vi "traitement cam 33.vi"() -> (11 "Couleur carré 11 (1,9)":string[](array[string]), 13 "Couleur carré 10  (1,8)":string[](array[string]), 14 "Couleur carré 4 (2,1)":string[](array[string]), 15 "Couleur carré 9 (1,7)":string[](array[string]), 16 "Couleur carré 3 (2,4)":string[](array[string]), 17 "Couleur carré 12 (1,4)":string[](array[string]), 18 "Couleur carré 2 (2,7)":string[](array[string]), 19 "Image Out":T2(plugin-control), 20 "Couleur carré 1 (2,8)":string[](array[string]), 22 "Couleur carré 5 (6,4)":string[](array[string]), 23 "Couleur carré 6 (6,1)":string[](array[string]), 24 "Couleur carré 7 (6,2)":string[](array[string]), 25 "Couleur carré 8 (6,3)":string[](array[string]), 27 "error out":errorcluster)   [LabVIEW 2019]
uses:
  <vilib>/vision/Classification.llb/IMAQ Classifier Read Options.ctl
  <vilib>/vision/NI_Vision_Development_Module.lvlib
panel:
  in  "ROI Carré 1":T1={"Global Rectangle"=[636, 369, 672, 405], "Contours"=[{"ID"=enum."External", "Type"=3, "Coordinates"=[636, 369, 672, 405]}]} {"Contours"."Type" items=["No Selection", "Point", "Line", "Rectangle", "Oval", "Polygon", "Freehand Region", "Annulus", "Unused2", "Unused3", "Broken Line", "Freehand Line", "Rotated Rectangle"]}
  in  "error in":errorcluster
  in  "ROI Carré 12":T1={"Global Rectangle"=[636, 369, 672, 405], "Contours"=[{"ID"=enum."External", "Type"=3, "Coordinates"=[636, 369, 672, 405]}]} {"Contours"."Type" items=["No Selection", "Point", "Line", "Rectangle", "Oval", "Polygon", "Freehand Region", "Annulus", "Unused2", "Unused3", "Broken Line", "Freehand Line", "Rotated Rectangle"]}
  in  "ROI Carré 11":T1={"Global Rectangle"=[636, 369, 672, 405], "Contours"=[{"ID"=enum."External", "Type"=3, "Coordinates"=[636, 369, 672, 405]}]} {"Contours"."Type" items=["No Selection", "Point", "Line", "Rectangle", "Oval", "Polygon", "Freehand Region", "Annulus", "Unused2", "Unused3", "Broken Line", "Freehand Line", "Rotated Rectangle"]}
  in  "ROI Carré 10":T1={"Global Rectangle"=[636, 369, 672, 405], "Contours"=[{"ID"=enum."External", "Type"=3, "Coordinates"=[636, 369, 672, 405]}]} {"Contours"."Type" items=["No Selection", "Point", "Line", "Rectangle", "Oval", "Polygon", "Freehand Region", "Annulus", "Unused2", "Unused3", "Broken Line", "Freehand Line", "Rotated Rectangle"]}
  in  "ROI Carré 9":T1={"Global Rectangle"=[636, 369, 672, 405], "Contours"=[{"ID"=enum."External", "Type"=3, "Coordinates"=[636, 369, 672, 405]}]} {"Contours"."Type" items=["No Selection", "Point", "Line", "Rectangle", "Oval", "Polygon", "Freehand Region", "Annulus", "Unused2", "Unused3", "Broken Line", "Freehand Line", "Rotated Rectangle"]}
  in  "ROI Carré 8":T1={"Global Rectangle"=[636, 369, 672, 405], "Contours"=[{"ID"=enum."External", "Type"=3, "Coordinates"=[636, 369, 672, 405]}]} {"Contours"."Type" items=["No Selection", "Point", "Line", "Rectangle", "Oval", "Polygon", "Freehand Region", "Annulus", "Unused2", "Unused3", "Broken Line", "Freehand Line", "Rotated Rectangle"]}
  in  "ROI Carré 7":T1={"Global Rectangle"=[636, 369, 672, 405], "Contours"=[{"ID"=enum."External", "Type"=3, "Coordinates"=[636, 369, 672, 405]}]} {"Contours"."Type" items=["No Selection", "Point", "Line", "Rectangle", "Oval", "Polygon", "Freehand Region", "Annulus", "Unused2", "Unused3", "Broken Line", "Freehand Line", "Rotated Rectangle"]}
  in  "ROI Carré 6":T1={"Global Rectangle"=[636, 369, 672, 405], "Contours"=[{"ID"=enum."External", "Type"=3, "Coordinates"=[636, 369, 672, 405]}]} {"Contours"."Type" items=["No Selection", "Point", "Line", "Rectangle", "Oval", "Polygon", "Freehand Region", "Annulus", "Unused2", "Unused3", "Broken Line", "Freehand Line", "Rotated Rectangle"]}
  in  "ROI Carré 5":T1={"Global Rectangle"=[636, 369, 672, 405], "Contours"=[{"ID"=enum."External", "Type"=3, "Coordinates"=[636, 369, 672, 405]}]} {"Contours"."Type" items=["No Selection", "Point", "Line", "Rectangle", "Oval", "Polygon", "Freehand Region", "Annulus", "Unused2", "Unused3", "Broken Line", "Freehand Line", "Rotated Rectangle"]}
  in  "ROI Carré 4":T1={"Global Rectangle"=[636, 369, 672, 405], "Contours"=[{"ID"=enum."External", "Type"=3, "Coordinates"=[636, 369, 672, 405]}]} {"Contours"."Type" items=["No Selection", "Point", "Line", "Rectangle", "Oval", "Polygon", "Freehand Region", "Annulus", "Unused2", "Unused3", "Broken Line", "Freehand Line", "Rotated Rectangle"]}
  in  "ROI Carré 3":T1={"Global Rectangle"=[636, 369, 672, 405], "Contours"=[{"ID"=enum."External", "Type"=3, "Coordinates"=[636, 369, 672, 405]}]} {"Contours"."Type" items=["No Selection", "Point", "Line", "Rectangle", "Oval", "Polygon", "Freehand Region", "Annulus", "Unused2", "Unused3", "Broken Line", "Freehand Line", "Rotated Rectangle"]}
  in  "ROI Carré 2":T1={"Global Rectangle"=[636, 369, 672, 405], "Contours"=[{"ID"=enum."External", "Type"=3, "Coordinates"=[636, 369, 672, 405]}]} {"Contours"."Type" items=["No Selection", "Point", "Line", "Rectangle", "Oval", "Polygon", "Freehand Region", "Annulus", "Unused2", "Unused3", "Broken Line", "Freehand Line", "Rotated Rectangle"]}
  # "C\nE\nN\nT\nR\nE\n\nJ\nA\nU\nN\nE\n\nBAS"
  # "C\nE\nN\nT\nR\nE\n\nV\nE\nR\nT\n\nG"
  # "C\nE\nN\nT\nR\nE\n\nR\nO\nU\nG\nE\n\nD"
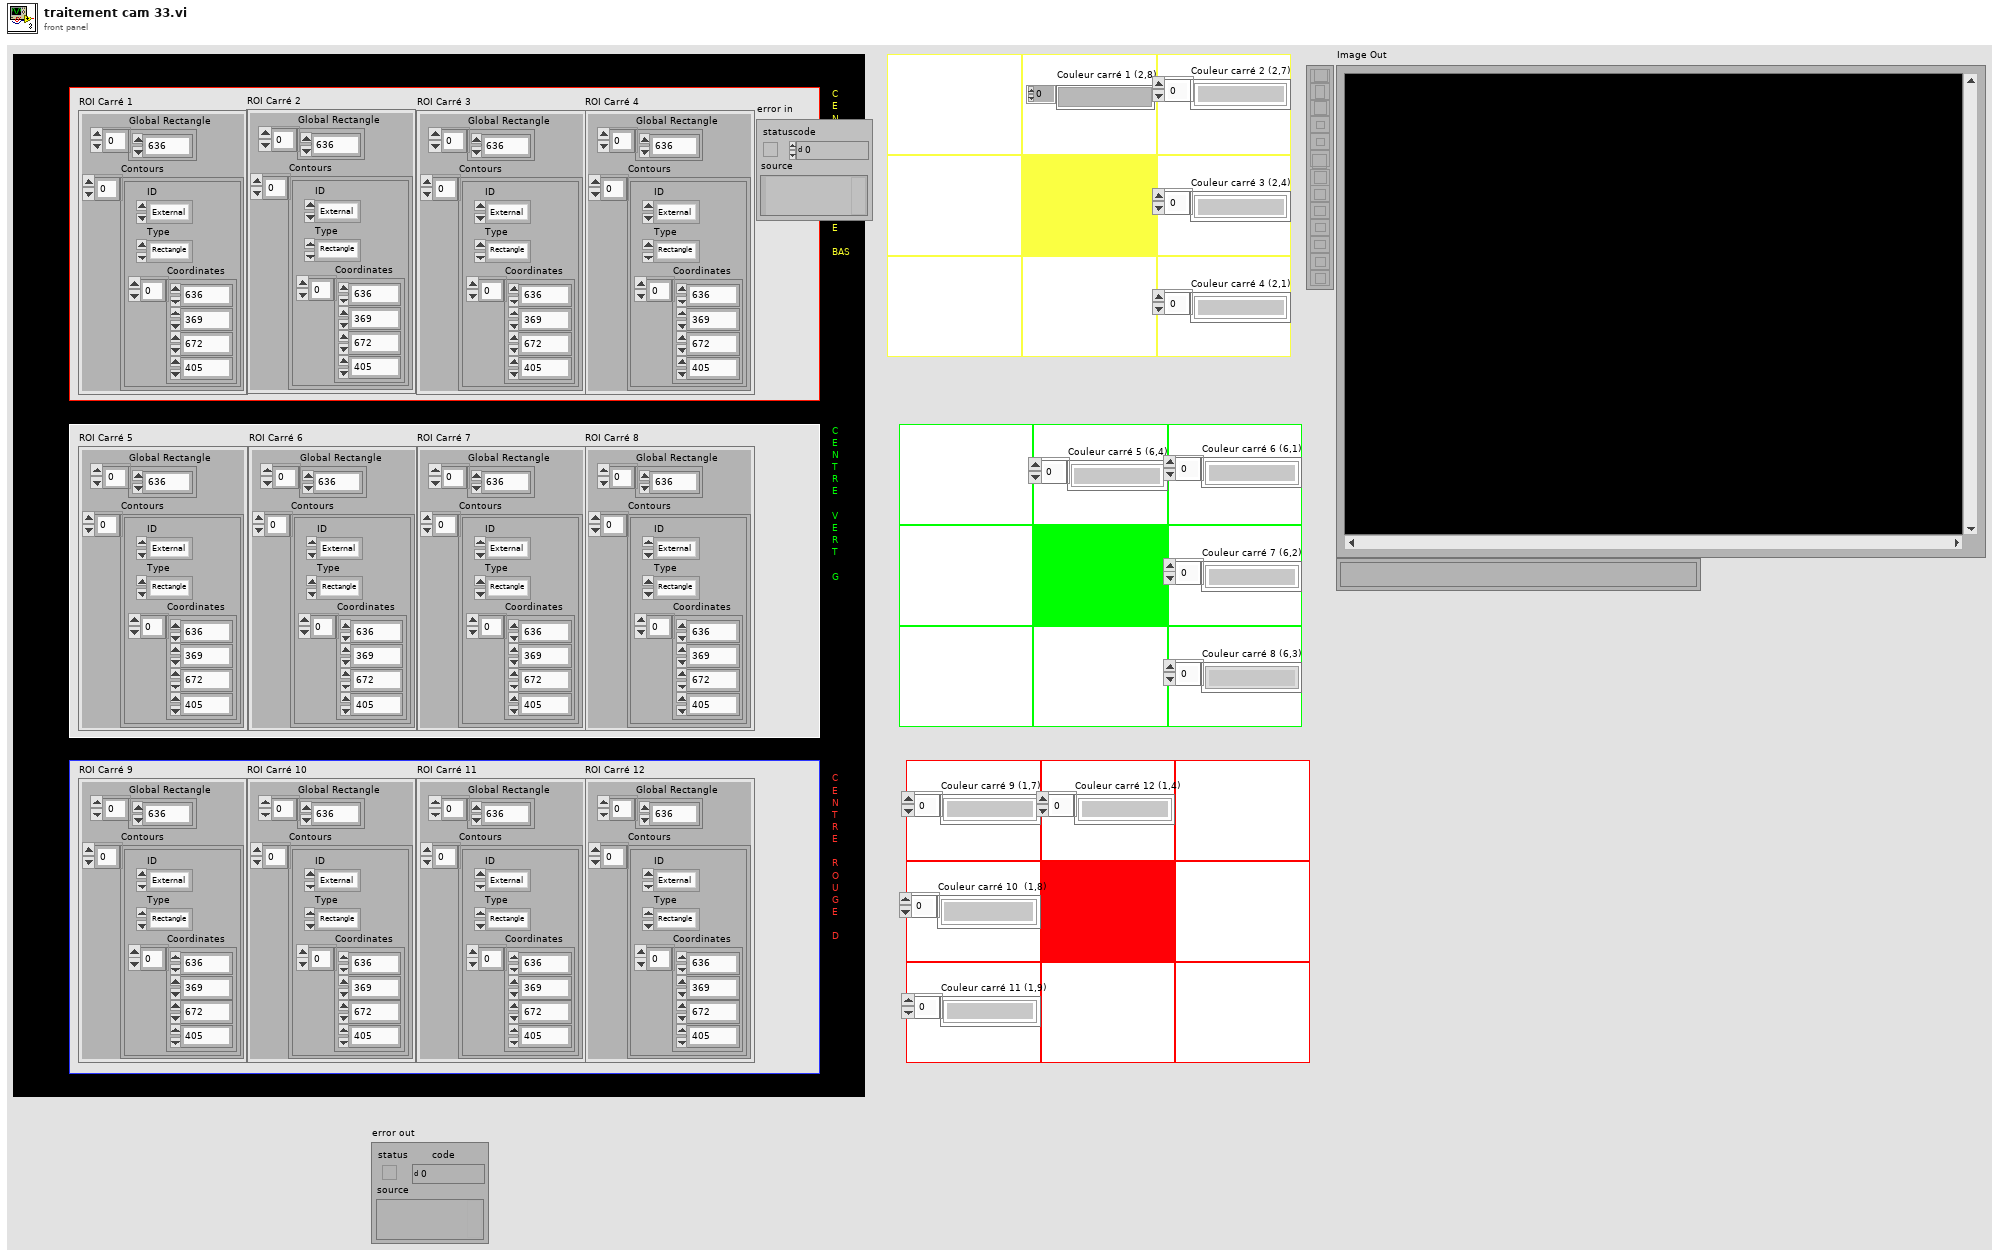
[diagram p1: front panel]
types:
  T1 = cluster{"Global Rectangle":i32[], "Contours":cluster{"ID":enum32{"External", "Internal"}, "Type":u32, "Coordinates":i32[]}[]}
  T2 = typedef "IMAQ Image.ctl" = refnum<image>
  T3 = typedef "IMAQ Classifier Read Options.ctl" = i32
  T4 = typedef "IMAQ Classifier Session.ctl" = refnum<k1>
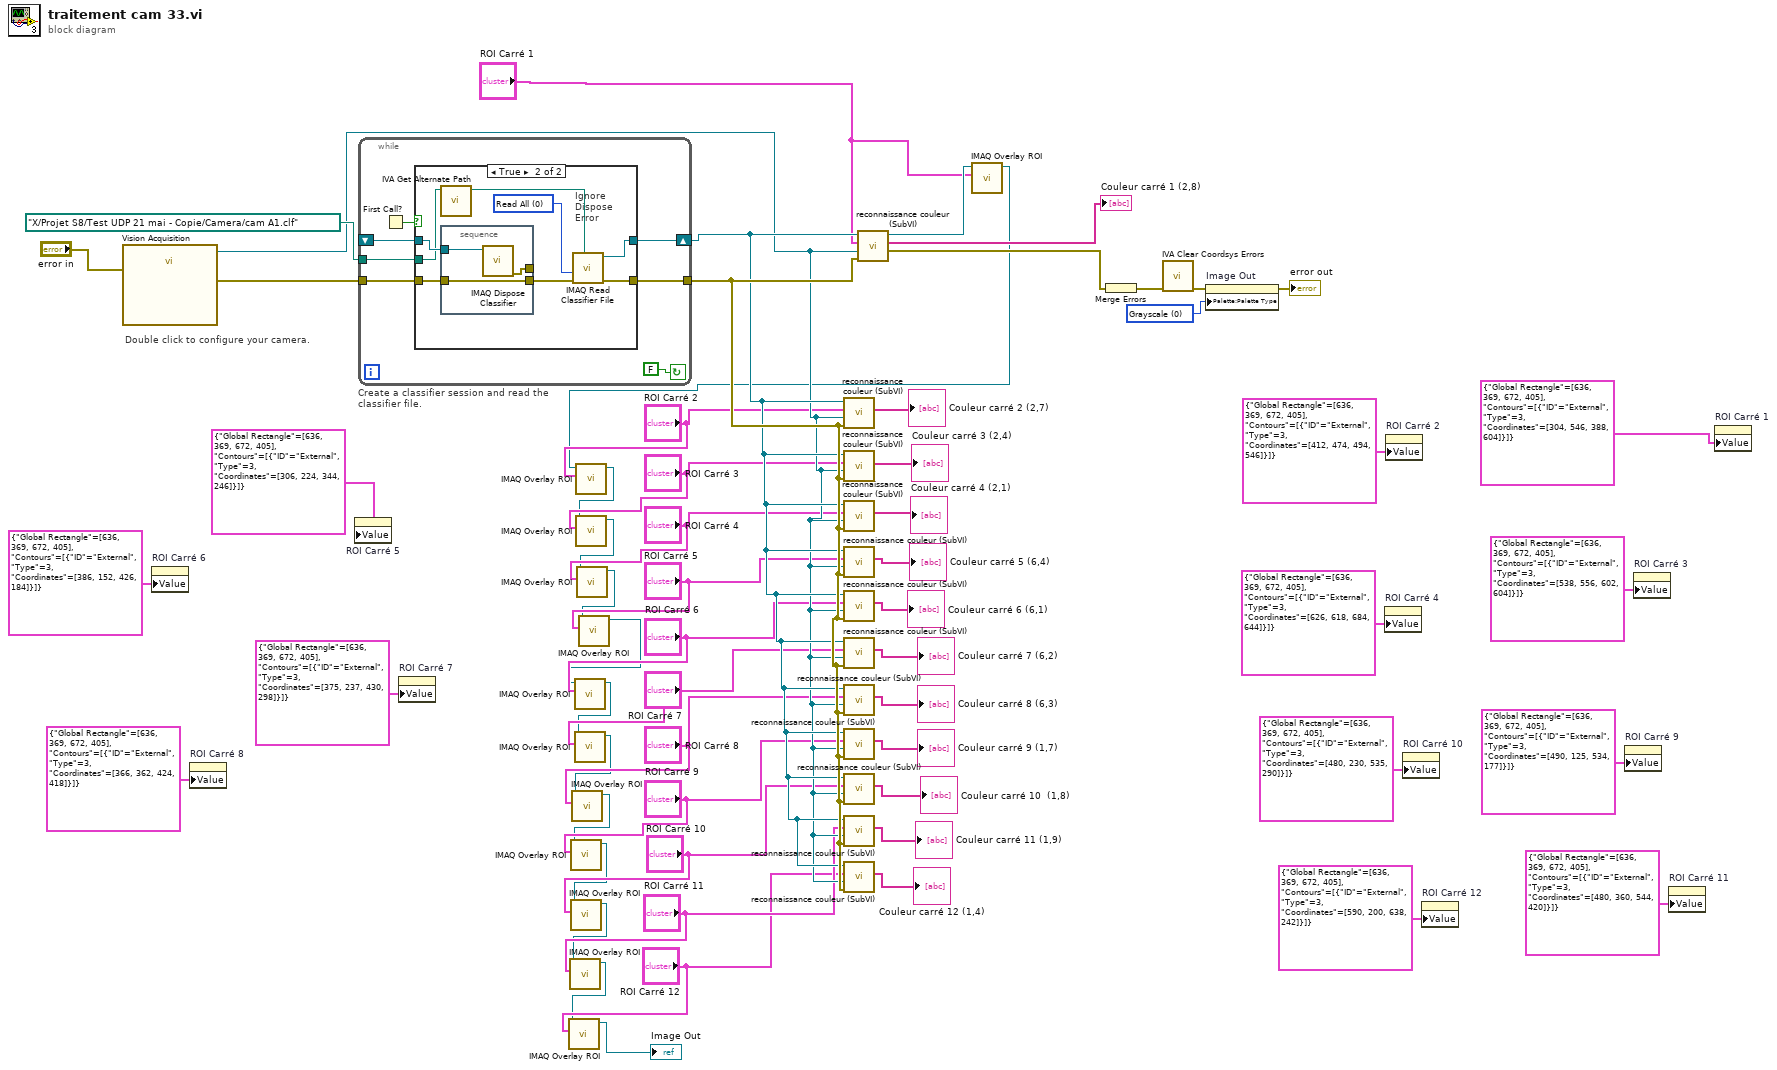
[diagram p0: block diagram]
diagram:
  w53 = u32 0 items=["Grayscale", "Binary", "Gradient", "Rainbow", "Temperature", "User Defined", "Binary 16 Bit", "Gradient 16 Bit", "Rainbow 16 Bit", "Temperature 16 Bit", "User Defined 16 Bit"] ("Palette Type")
  # "Double click to configure your camera."
  n1 = call "Vision Acquisition"("error in"="error in") -> ("Image Out"=w39:T2, "error out"=w58:errorcluster)  [unwired: 25 in]
  n2 = property on="ROI Carré 6" class="Clust (strict)"("Value"=T1 {"Global Rectangle"=[636, 369, 672, 405], "Contours"=[{"ID"=enum."External", "Type"=3, "Coordinates"=[386, 152, 426, 184]}]} ("ROI Carré 6")) -> ()  [unwired: 2 in, 2 out]
  n3 = property on="ROI Carré 8" class="Clust (strict)"("Value"=T1 {"Global Rectangle"=[636, 369, 672, 405], "Contours"=[{"ID"=enum."External", "Type"=3, "Coordinates"=[366, 362, 424, 418]}]} ("ROI Carré 8")) -> ()  [unwired: 2 in, 2 out]
  n4 = property on="ROI Carré 5" class="Clust (strict)"("Value"=T1 {"Global Rectangle"=[636, 369, 672, 405], "Contours"=[{"ID"=enum."External", "Type"=3, "Coordinates"=[306, 224, 344, 246]}]} ("ROI Carré 5")) -> ()  [unwired: 2 in, 2 out]
  n5 = while "Create a classifier session and read the classifier file." {
    shift-right: [w67] -> w50
    shift-left: _ -> [w66]
    tunnel: w58 -> [w64]
    tunnel: [w63] -> w51
    tunnel: path "X:/Projet S8/Test UDP 21 mai - Copie/Camera/cam A1.clf" ("File Path") -> [w62]
    stop <- FALSE continue-if-true
    n6 = First Call?() -> (First Call?: T/F=w61:bool)
    n7 = case shown="True" w61 {
      tunnel: [w69 w76] -> w67
      tunnel: w66 -> [w69 w74]
      tunnel: w64 -> [w68 w73]
      tunnel: [w68 w75] -> w63
      tunnel: w62 -> [_ w71]
      frame False {
      }
      frame True {
        w77 = T3 0 items=["Read All", "Add Samples, Do Not Change Options", "Read Options, Do Not Add Samples"] ("Read Options")
        # "Ignore Dispose Error"
        n8 = call <vilib>:"IVA Get Alternate Path.vi"("Path In"=w71) -> ("Path Out"=w70:path)  [unwired: 10 out]
        n9 = stacked-sequence {
          tunnel: w74 -> [w80]
          tunnel: w73 -> [w79]
          tunnel: [w79] -> w72
          tunnel: [w78] -> _
          frame #0 {
            n10 = call "IMAQ Dispose Classifier"("Classifier Session"=w80) -> ("error out"=w78:errorcluster)  [unwired: 1 in, 9 out]
          }
        }
        n11 = call "IMAQ Read Classifier File"("File Path"=w70, "error in (no error)"=w72, "Read Options"=w77) -> ("error out"=w75:errorcluster, "Classifier Session"=w76:T4)  [unwired: 1 in, 6 out]
      }
    }
  }
  n12 = property on="ROI Carré 7" class="Clust (strict)"("Value"=T1 {"Global Rectangle"=[636, 369, 672, 405], "Contours"=[{"ID"=enum."External", "Type"=3, "Coordinates"=[375, 237, 430, 298]}]} ("ROI Carré 7")) -> ()  [unwired: 2 in, 2 out]
  n13 = call "reconnaissance couleur (SubVI).vi"("error in (no error)"=w51, "Image Out in"=w39, "ROI Descriptor (Color Classification 1)"="ROI Carré 2", "Refnum in"=w50) -> ("Array 2"=→"Couleur carré 2 (2,7)":string[])  [unwired: 5 in, 2 out]
  n14 = call "reconnaissance couleur (SubVI).vi"("error in (no error)"=w51, "Image Out in"=w39, "ROI Descriptor (Color Classification 1)"="ROI Carré 3", "Refnum in"=w50) -> ("Array 2"=→"Couleur carré 3 (2,4)":string[])  [unwired: 5 in, 2 out]
  n15 = call "reconnaissance couleur (SubVI).vi"("error in (no error)"=w51, "Image Out in"=w39, "ROI Descriptor (Color Classification 1)"="ROI Carré 4", "Refnum in"=w50) -> ("Array 2"=→"Couleur carré 4 (2,1)":string[])  [unwired: 5 in, 2 out]
  n16 = call "reconnaissance couleur (SubVI).vi"("error in (no error)"=w51, "Image Out in"=w39, "ROI Descriptor (Color Classification 1)"="ROI Carré 5", "Refnum in"=w50) -> ("Array 2"=→"Couleur carré 5 (6,4)":string[])  [unwired: 5 in, 2 out]
  n17 = call "reconnaissance couleur (SubVI).vi"("error in (no error)"=w51, "Image Out in"=w39, "ROI Descriptor (Color Classification 1)"="ROI Carré 6", "Refnum in"=w50) -> ("Array 2"=→"Couleur carré 6 (6,1)":string[])  [unwired: 5 in, 2 out]
  n18 = call "reconnaissance couleur (SubVI).vi"("error in (no error)"=w51, "Image Out in"=w39, "ROI Descriptor (Color Classification 1)"="ROI Carré 7", "Refnum in"=w50) -> ("Array 2"=→"Couleur carré 7 (6,2)":string[])  [unwired: 5 in, 2 out]
  n19 = call "reconnaissance couleur (SubVI).vi"("error in (no error)"=w51, "Image Out in"=w39, "ROI Descriptor (Color Classification 1)"="ROI Carré 8", "Refnum in"=w50) -> ("Array 2"=→"Couleur carré 8 (6,3)":string[])  [unwired: 5 in, 2 out]
  n20 = call "reconnaissance couleur (SubVI).vi"("error in (no error)"=w51, "Image Out in"=w39, "ROI Descriptor (Color Classification 1)"="ROI Carré 9", "Refnum in"=w50) -> ("Array 2"=→"Couleur carré 9 (1,7)":string[])  [unwired: 5 in, 2 out]
  n21 = call "reconnaissance couleur (SubVI).vi"("error in (no error)"=w51, "Image Out in"=w39, "ROI Descriptor (Color Classification 1)"="ROI Carré 10", "Refnum in"=w50) -> ("Array 2"=→"Couleur carré 10  (1,8)":string[])  [unwired: 5 in, 2 out]
  n22 = call "reconnaissance couleur (SubVI).vi"("error in (no error)"=w51, "Image Out in"=w39, "ROI Descriptor (Color Classification 1)"="ROI Carré 11", "Refnum in"=w50) -> ("Array 2"=→"Couleur carré 11 (1,9)":string[])  [unwired: 5 in, 2 out]
  n23 = call "reconnaissance couleur (SubVI).vi"("error in (no error)"=w51, "Image Out in"=w39, "ROI Descriptor (Color Classification 1)"="ROI Carré 12", "Refnum in"=w50) -> ("Array 2"=→"Couleur carré 12 (1,4)":string[])  [unwired: 5 in, 2 out]
  n24 = call "reconnaissance couleur (SubVI).vi"("error in (no error)"=w51, "Image Out in"=w39, "ROI Descriptor (Color Classification 1)"="ROI Carré 1", "Refnum in"=w50) -> ("Array"=w57:errorcluster[], "Array 2"=→"Couleur carré 1 (2,8)":string[], "Refnum out"=w38:T2)  [unwired: 5 in]
  n25 = call "IMAQ Overlay ROI"("ROI Descriptor"="ROI Carré 1", "Image"=w38) -> ("Image Out"=w36:T2)  [unwired: 8 in, 1 out]
  n26 = call "IMAQ Overlay ROI"("ROI Descriptor"="ROI Carré 2", "Image"=w36) -> ("Image Out"=w25:T2)  [unwired: 8 in, 1 out]
  n27 = call "IMAQ Overlay ROI"("ROI Descriptor"="ROI Carré 3", "Image"=w25) -> ("Image Out"=w24:T2)  [unwired: 8 in, 1 out]
  n28 = call "IMAQ Overlay ROI"("ROI Descriptor"="ROI Carré 4", "Image"=w24) -> ("Image Out"=w23:T2)  [unwired: 8 in, 1 out]
  n29 = call "IMAQ Overlay ROI"("ROI Descriptor"="ROI Carré 5", "Image"=w23) -> ("Image Out"=w22:T2)  [unwired: 8 in, 1 out]
  n30 = call "IMAQ Overlay ROI"("ROI Descriptor"="ROI Carré 6", "Image"=w22) -> ("Image Out"=w21:T2)  [unwired: 8 in, 1 out]
  n31 = call "IMAQ Overlay ROI"("ROI Descriptor"="ROI Carré 7", "Image"=w21) -> ("Image Out"=w20:T2)  [unwired: 8 in, 1 out]
  n32 = call "IMAQ Overlay ROI"("ROI Descriptor"="ROI Carré 8", "Image"=w20) -> ("Image Out"=w19:T2)  [unwired: 8 in, 1 out]
  n33 = call "IMAQ Overlay ROI"("ROI Descriptor"="ROI Carré 9", "Image"=w19) -> ("Image Out"=w18:T2)  [unwired: 8 in, 1 out]
  n34 = call "IMAQ Overlay ROI"("ROI Descriptor"="ROI Carré 10", "Image"=w18) -> ("Image Out"=w17:T2)  [unwired: 8 in, 1 out]
  n35 = call "IMAQ Overlay ROI"("ROI Descriptor"="ROI Carré 11", "Image"=w17) -> ("Image Out"=w16:T2)  [unwired: 8 in, 1 out]
  n36 = call "IMAQ Overlay ROI"("ROI Descriptor"="ROI Carré 12", "Image"=w16) -> ("Image Out"=→"Image Out":T2)  [unwired: 8 in, 1 out]
  n37 = Merge Errors(w57) -> (w56:errorcluster)
  n38 = call <vilib>:"IVA Clear Coordsys Errors.vi"("error in (no error)"=w56) -> ("error out"=w55:errorcluster)  [unwired: 10 in]
  n39 = property on="Image Out" class="ImageControl"(error in=w55, "Palette:Palette Type"=w53) -> (error out=→"error out":errorcluster)  [unwired: 1 in, 1 out]
  n40 = property on="ROI Carré 4" class="Clust (strict)"("Value"=T1 {"Global Rectangle"=[636, 369, 672, 405], "Contours"=[{"ID"=enum."External", "Type"=3, "Coordinates"=[626, 618, 684, 644]}]} ("ROI Carré 4")) -> ()  [unwired: 2 in, 2 out]
  n41 = property on="ROI Carré 2" class="Clust (strict)"("Value"=T1 {"Global Rectangle"=[636, 369, 672, 405], "Contours"=[{"ID"=enum."External", "Type"=3, "Coordinates"=[412, 474, 494, 546]}]} ("ROI Carré 2")) -> ()  [unwired: 2 in, 2 out]
  n42 = property on="ROI Carré 10" class="Clust (strict)"("Value"=T1 {"Global Rectangle"=[636, 369, 672, 405], "Contours"=[{"ID"=enum."External", "Type"=3, "Coordinates"=[480, 230, 535, 290]}]} ("ROI Carré 10")) -> ()  [unwired: 2 in, 2 out]
  n43 = property on="ROI Carré 12" class="Clust (strict)"("Value"=T1 {"Global Rectangle"=[636, 369, 672, 405], "Contours"=[{"ID"=enum."External", "Type"=3, "Coordinates"=[590, 200, 638, 242]}]} ("ROI Carré 12")) -> ()  [unwired: 2 in, 2 out]
  n44 = property on="ROI Carré 9" class="Clust (strict)"("Value"=T1 {"Global Rectangle"=[636, 369, 672, 405], "Contours"=[{"ID"=enum."External", "Type"=3, "Coordinates"=[490, 125, 534, 177]}]} ("ROI Carré 9")) -> ()  [unwired: 2 in, 2 out]
  n45 = property on="ROI Carré 3" class="Clust (strict)"("Value"=T1 {"Global Rectangle"=[636, 369, 672, 405], "Contours"=[{"ID"=enum."External", "Type"=3, "Coordinates"=[538, 556, 602, 604]}]} ("ROI Carré 3")) -> ()  [unwired: 2 in, 2 out]
  n46 = property on="ROI Carré 11" class="Clust (strict)"("Value"=T1 {"Global Rectangle"=[636, 369, 672, 405], "Contours"=[{"ID"=enum."External", "Type"=3, "Coordinates"=[480, 360, 544, 420]}]} ("ROI Carré 11")) -> ()  [unwired: 2 in, 2 out]
  n47 = property on="ROI Carré 1" class="Clust (strict)"("Value"=T1 {"Global Rectangle"=[636, 369, 672, 405], "Contours"=[{"ID"=enum."External", "Type"=3, "Coordinates"=[304, 546, 388, 604]}]} ("ROI Carré 1")) -> ()  [unwired: 2 in, 2 out]
